vi "Start Stream.vi"(8 "error in (no error)":errorcluster, 10 "Camera Settings":T1={"Exposure Time (ms)"=100.0, "Binning"=enum."2x2", "Scan Mode"=0, "Frames to Acquire"=1000.0, "Pixel Correction"=FALSE, "Frames to Skip"=0, "File Path"=path "", "Duty cycle"=0.0, "ALEX"=FALSE, "Shutter Enable"=[], "fluidics trigger frame"=0, "Bit Depth"=0, "Image Width (px)"=0, "Image Height (px)"=0, "Horizontal Offset (px)"=0, "Vertical Offset (px)"=0} {"fluidics trigger frame" max=60000 step=1; "Exposure Time (ms)" min=1.0 max=10000.0 step=1.0}, 11 "Photometrics Camera in":refnum<class "Photometrics Camera.lvclass">) -> (0 "error out":errorcluster, 3 "Photometrics Camera out":refnum<class "Photometrics Camera.lvclass">)   [LabVIEW 2022 SP3, in "Photometrics Camera.lvlib" / "Photometrics Camera.lvclass"]
uses:
  Photometrics Camera.lvclass
  Resources/Type Defs/Camera Settings.ctl
  Resources/Type Defs/Camera Type.ctl
  9801741b-1c9a-4d7a-a0e8-766f0520d7c1.vi
  C:/FlashGordon/Development/dll/PVCamNET.dll
  dll/PVCamNET.dll
  Camera/Camera.lvclass
panel:
  out "name":string
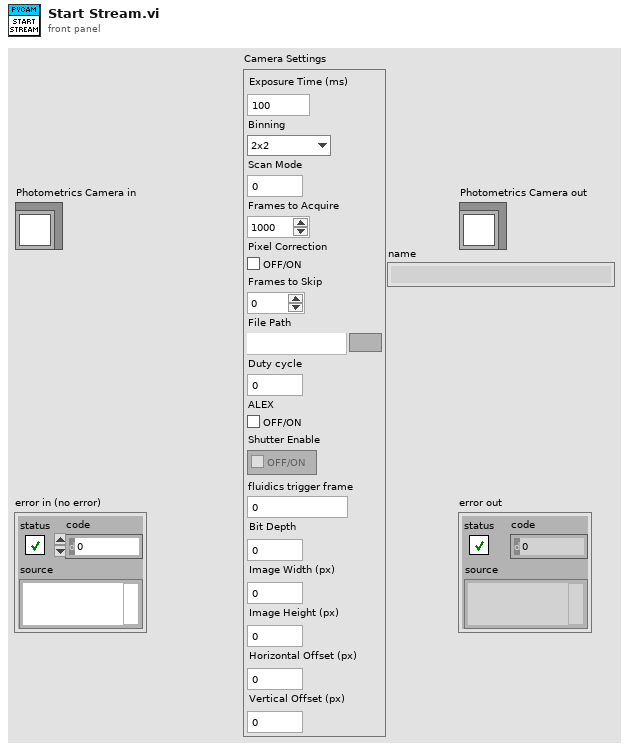
[diagram p1: front panel]
types:
  T1 = typedef "Camera Settings.ctl" = cluster{"Exposure Time (ms)":dbl, "Binning":enum16{"1x1", "2x2", "4x4"}, "Scan Mode":i32, "Frames to Acquire":dbl, "Pixel Correction":bool, "Frames to Skip":u32, "File Path":path, "Duty cycle":dbl, "ALEX":bool, "Shutter Enable":bool[], "fluidics trigger frame":u16, "Bit Depth":u16, "Image Width (px)":u16, "Image Height (px)":u16, "Horizontal Offset (px)":u16, "Vertical Offset (px)":u16}
  T2 = typedef "Camera Type.ctl" = enum16{"Hamamatsu", "Andor", "Photometrics"}
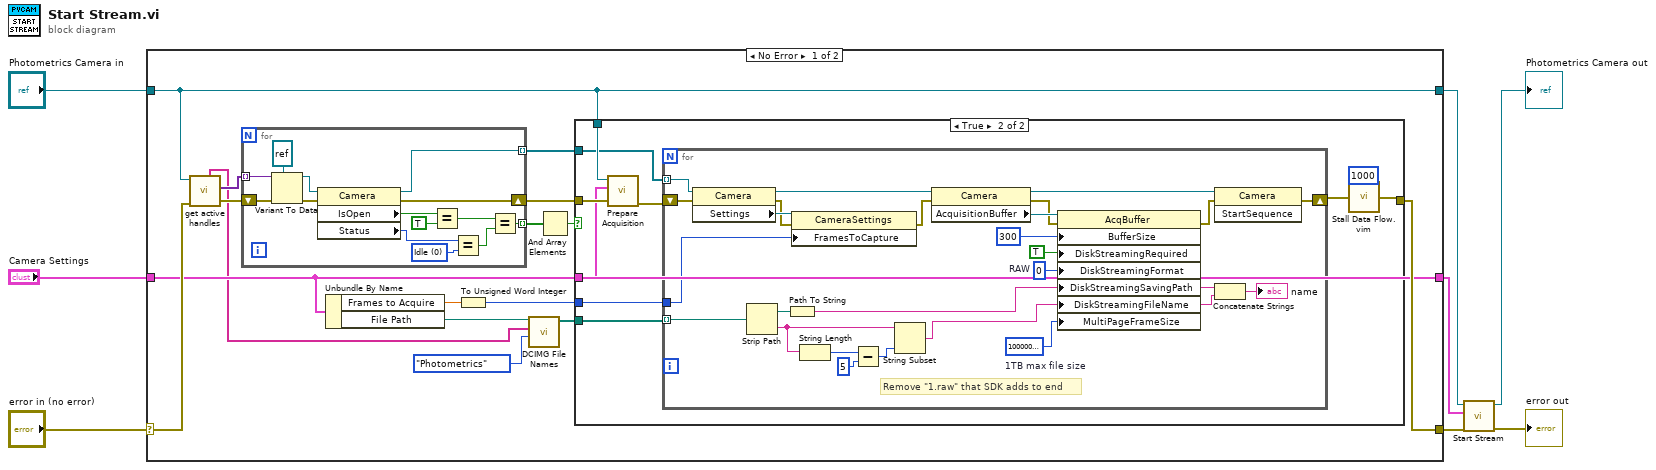
[diagram p0: block diagram]
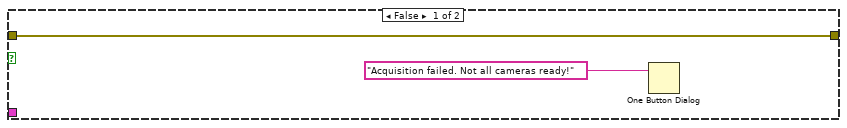
[diagram p2: hidden frame]
diagram:
  n1 = case shown="No Error" "error in (no error)" {
    selector: "error in (no error)" -> [w18 w78]
    tunnel: [w17 w78] -> w5
    tunnel: "Photometrics Camera in" -> [w16 w77]
    tunnel: [w16 w77] -> w3
    tunnel: "Camera Settings" -> [w15 w76]
    tunnel: [w15 w76] -> w1
    frame No Error {
      n2 = call-dynamic "get active handles.vi"("error in (no error)"=w18, "Camera in"=w16) -> ("error out"=w21:errorcluster, "Handles"=w20:variant[], "Camera Names"=w11:string[])  [unwired: 5 in, 2 out]
      n3 = for {
        tunnel: [w69] -> w23 mode=indexing
        tunnel: w20 -> [w66] mode=indexing
        shift-right: [w68] -> w24
        shift-left: w21 -> [w65]
        tunnel: [w67] -> w19 mode=indexing
        w74 = 0 items=["Idle", "Capturing"] ("Status")
        n4 = Variant To Data(error in=w65, type=refnum<k24> refnum ("reference out"), Variant=w66) -> (data=w63:refnum<k24>, error out=w64:errorcluster)
        n5 = property class="Camera"(reference=w63, error in=w64) -> (reference out=w67:refnum<k24>, error out=w68:errorcluster, "IsOpen"=w73:bool, "Status"=w75:i32)
        n6 = Equal?(x=w73, y=TRUE) -> (x = y?=w71:bool)
        n7 = Equal?(x=w75, y=w74) -> (x = y?=w70:bool)
        n8 = Equal?(x=w71, y=w70) -> (x = y?=w69:bool)
      }
      n9 = Unbundle By Name(w15) -> ("Frames to Acquire"=w14:dbl, "File Path"=w10:path)
      n10 = To Unsigned Word Integer(number=w14) -> (unsigned 16bit integer=w13:u16)
      n11 = call "DCIMG File Names.vi"("Camera Type"=Camera_Type."Photometrics", "Channel Names"=w11, "TIFF File Path"=w10) -> ("DCIMG Files"=w9:path[])  [unwired: 8 in]
      n12 = And Array Elements(Boolean array=w23) -> (logical AND=w22:bool)
      n13 = case shown="True" w22 {
        tunnel: [w26 w28] -> w17
        tunnel: w24 -> [w26 w36]
        tunnel: w16 -> [_ w34]
        tunnel: w15 -> [_ w32]
        tunnel: w19 -> [_ w33]
        tunnel: w13 -> [_ w31]
        tunnel: w9 -> [_ w27]
        frame False {
          n14 = One Button Dialog(message="Acquisition failed. Not all cameras ready!") -> ()  [unwired: 1 in, 1 out]
        }
        frame True {
          n15 = call-dynamic "Prepare Acquisition.vi"("error in (no error)"=w36, "Camera Settings"=w32, "Photometrics Camera in"=w34) -> ("error out"=w35:errorcluster)  [unwired: 7 in, 1 out]
          n16 = for {
            tunnel: w33 -> [w56] mode=indexing
            shift-right: [w61] -> w29
            shift-left: w35 -> [w55]
            tunnel: w31 -> [w50]
            tunnel: w27 -> [w42] mode=indexing
            w45 = u64 1000000000000  # 1TB max file size
            w46 = u32 0  # RAW
            # "Remove \"1.raw\" that SDK adds to end"
            n17 = property class="Camera"(reference=w56, error in=w55) -> (reference out=w52:refnum<k24>, error out=w53:errorcluster, "Settings"=w54:refnum<k24>)
            n18 = Strip Path(path=w42) -> (stripped path=w49:path, name=w40:string)
            n19 = Path To String(path=w49) -> (string=w43:string)
            n20 = property class="CameraSettings"(reference=w54, error in=w53, "FramesToCapture"=w50) -> (error out=w51:errorcluster)  [unwired: 1 out]
            n21 = String Length(string=w40) -> (length=w38:i32)
            n22 = Subtract(x=w38, y=5) -> (x-y=w39:i32)
            n23 = String Subset(string=w40, length (rest)=w39) -> (substring=w41:string)  [unwired: 1 in]
            n24 = property class="Camera"(reference=w52, error in=w51) -> (reference out=w60:refnum<k24>, error out=w58:errorcluster, "AcquisitionBuffer"=w59:refnum<k24>)
            n25 = property class="AcqBuffer"(reference=w59, error in=w58, "BufferSize"=u32 300, "DiskStreamingRequired"=TRUE ("UseScaling"), "DiskStreamingFormat"=w46, "DiskStreamingSavingPath"=w43, "DiskStreamingFileName"=w41, "MultiPageFrameSize"=w45) -> (error out=w57:errorcluster)  [unwired: 1 out]
            n26 = invoke class="Camera" method="StartSequence"(reference=w60, error in=w57) -> (error out=w61:errorcluster)  [unwired: 1 in, 2 out]
            n27 = Concatenate Strings(w43, w41) -> (→"name":string)
          }
          n28 = call "Stall Data Flow.vim"("value in"=w29, "milliseconds to wait"=u32 1000) -> ("value out"=w28:errorcluster)  [unwired: 1 out]
        }
      }
    }
    frame Error {
    }
  }
  n29 = call-parent "Start Stream.vi"("error in (no error)"=w5, "Camera Settings"=w1, "Camera in"=w3) -> ("error out"=→"error out":errorcluster, "Camera out"=→"Photometrics Camera out":refnum<class "Photometrics Camera.lvclass">)  [unwired: 7 in]
